vi "autoqueue.vi"(0 "cluster":T3, 1 "output cluster":T2, 3 "Cluster":cluster{"1":bool, "2":bool}, 4 "Report Data.Degree":dbl[][](array[numeric]), 5 "1to4":T1, 6 "milliseconds to wait":u32=100, 7 "path?":bool, 8 "milliseconds to wait 2":u32=100, 11 "error out":errorcluster, 12 "reference":refnum<vi>, 13 "Str Refnum":refnum<vi>, 14 "reference 2":refnum<vi>) -> (15 "error out 2":errorcluster)   [LabVIEW 2015]
uses:
  Typedef/Inst. Queue.ctl
  Typedef/State.ctl
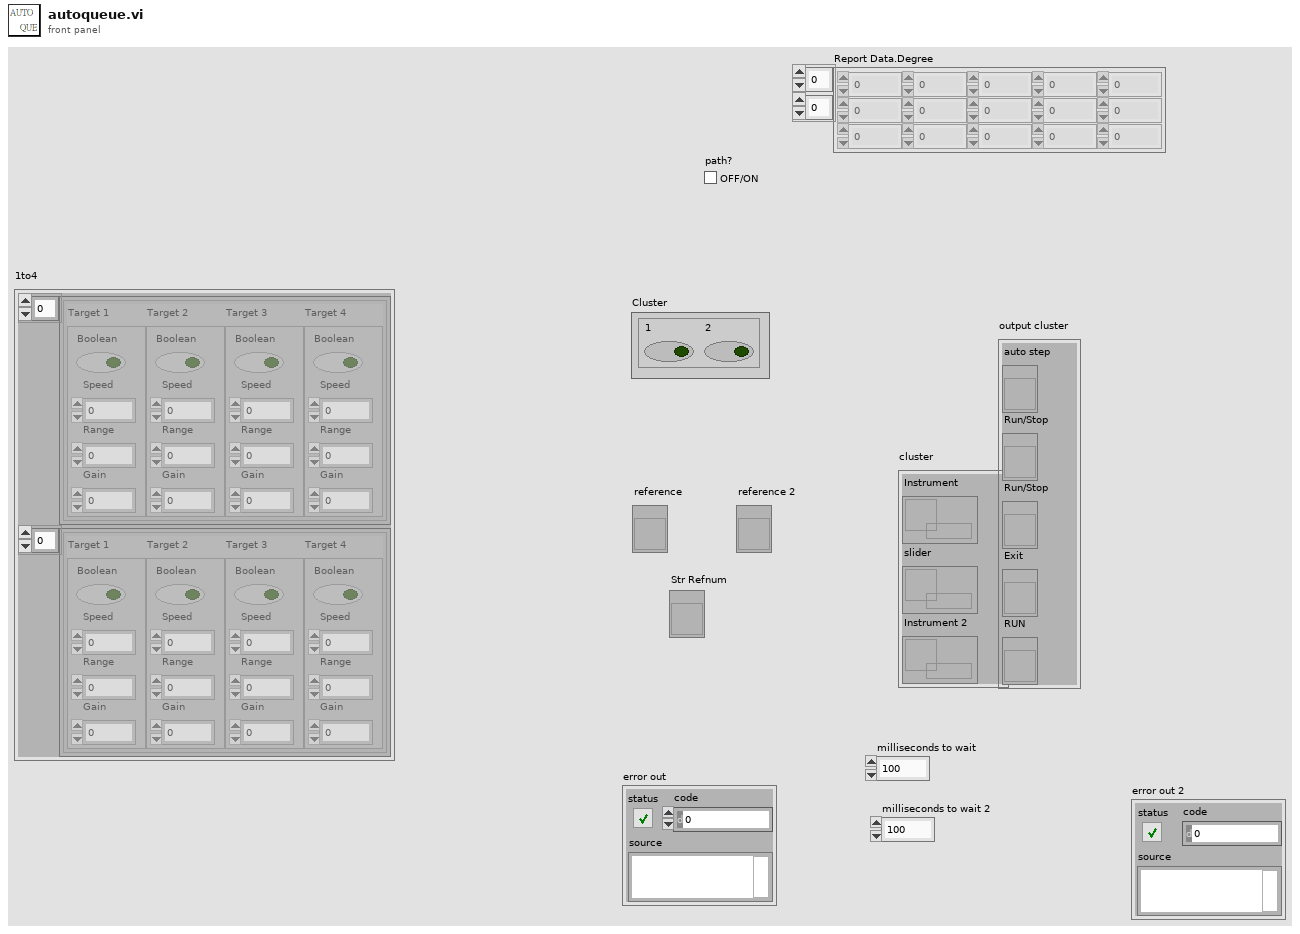
[diagram p1: front panel]
types:
  T1 = cluster{cluster{"Target 1":cluster{"Boolean":bool, "Speed":dbl, "Range":dbl, "Gain":dbl}, "Target 2":cluster{"Boolean":bool, "Speed":dbl, "Range":dbl, "Gain":dbl}, "Target 3":cluster{"Boolean":bool, "Speed":dbl, "Range":dbl, "Gain":dbl}, "Target 4":cluster{"Boolean":bool, "Speed":dbl, "Range":dbl, "Gain":dbl}}[], cluster{"Target 1":cluster{"Boolean":bool, "Speed":dbl, "Range":dbl, "Gain":dbl}, "Target 2":cluster{"Boolean":bool, "Speed":dbl, "Range":dbl, "Gain":dbl}, "Target 3":cluster{"Boolean":bool, "Speed":dbl, "Range":dbl, "Gain":dbl}, "Target 4":cluster{"Boolean":bool, "Speed":dbl, "Range":dbl, "Gain":dbl}}[]}
  T2 = cluster{"auto step":refnum<vi>, "Run/Stop":refnum<vi>, "Run/Stop":refnum<vi>, "Exit":refnum<vi>, "RUN":refnum<vi>}
  T3 = cluster{"Instrument":refnum<queue>, "slider":refnum<queue>, "Instrument 2":refnum<queue>}
  T4 = typedef "Inst. Queue.ctl" = cluster{enum16{"auto mode", "Idle", "Inst. Connect", "£m Data", "Inst. Update", "Freq. (GHz)", "rx att", "GTX (dB)", "GRX (dB)", "Range Trim(m)", "Gain Trim (dB)", "Distance to RUT", "Mapping", "Convert", "RF ON/OFF", "Run", "Direct Program", "Stop", "Dynamic", "dyset", "Exit"}, "variant":variant}
  T5 = cluster{"Target 1":cluster{"Boolean":bool, "Speed":dbl, "Range":dbl, "Gain":dbl}, "Target 2":cluster{"Boolean":bool, "Speed":dbl, "Range":dbl, "Gain":dbl}, "Target 3":cluster{"Boolean":bool, "Speed":dbl, "Range":dbl, "Gain":dbl}, "Target 4":cluster{"Boolean":bool, "Speed":dbl, "Range":dbl, "Gain":dbl}}[]
  T6 = typedef "State.ctl" = enum16{"Idle", "Initial", "Update", "get angle", "Axis", "Connect", "Creep", "Speed", "Distance", "Move Method", "Move Mode", "Direct of Movement", "Initail Speed", "Sramp", "Normal Open", "Acceleration", "Deceleration", "Angle", "Move&Rotate", "Rotate", "Rotate_2", "Return to Origin", "Move", "Inching", "Return to Zero", "Return to Middle", "Go to Step1", "Go to Step2", "Go to Step3", "Initial to Y Step", "Select Speed", "auto mode", "Stop", "reset xy", "reset ant", "set speed", "Exit"}
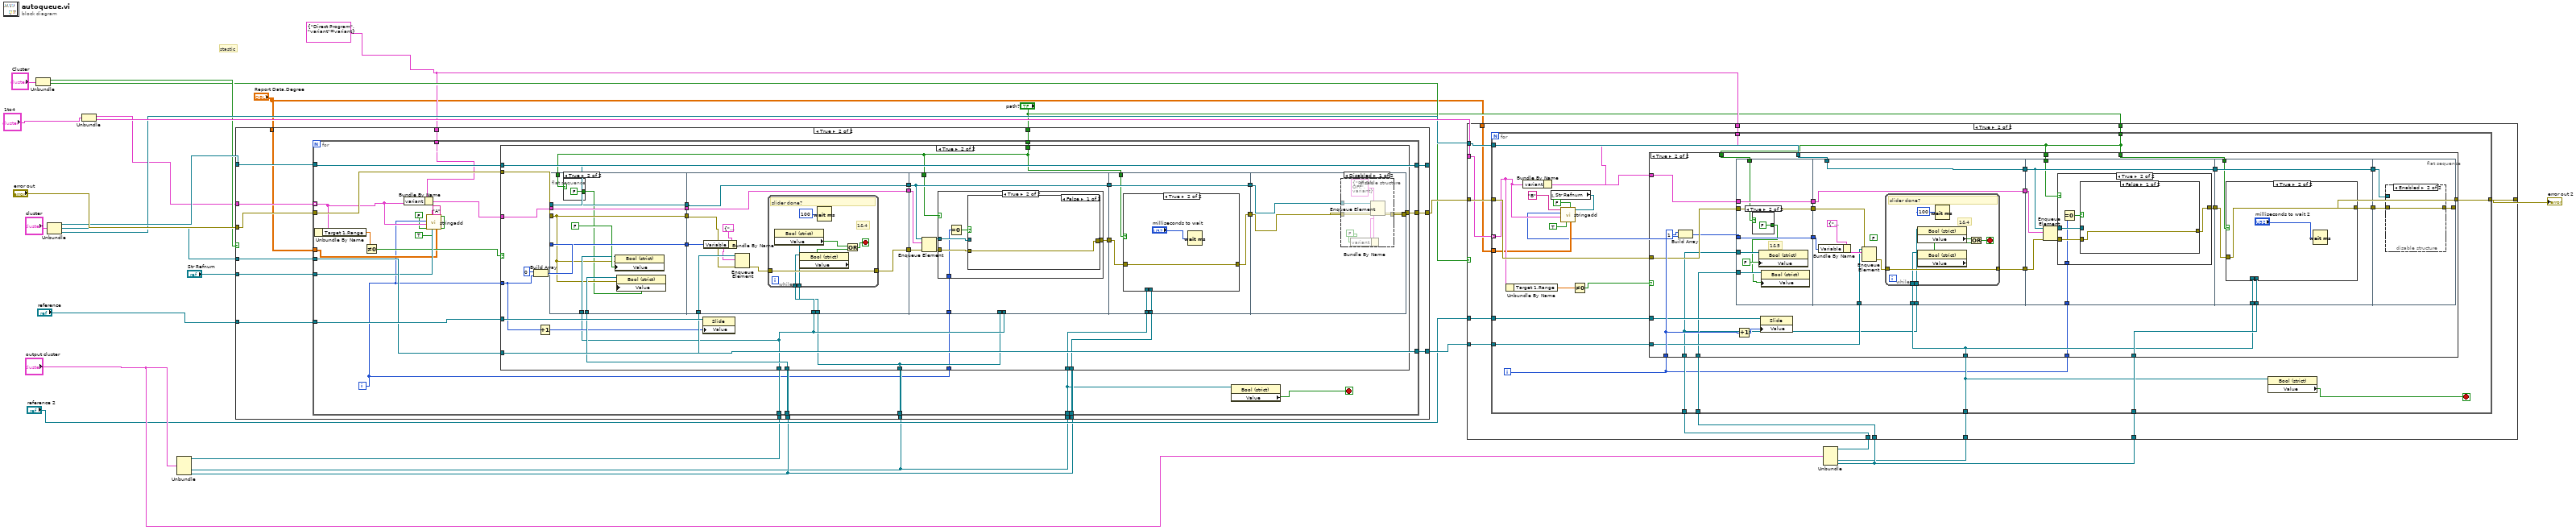
[diagram p0: block diagram]
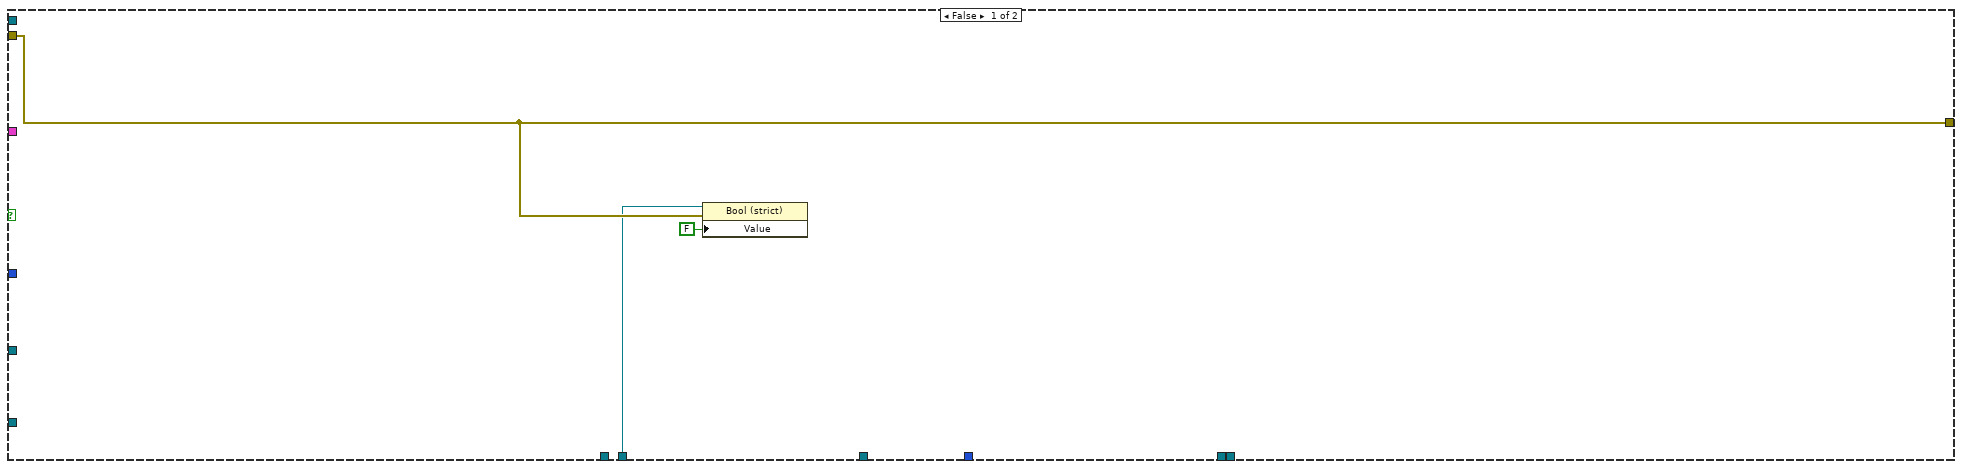
[diagram p3: hidden frame]
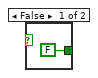
[diagram p4: hidden frame]
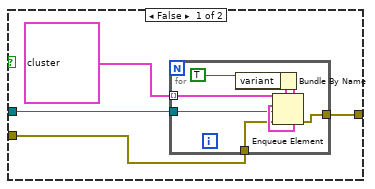
[diagram p5: hidden frame]
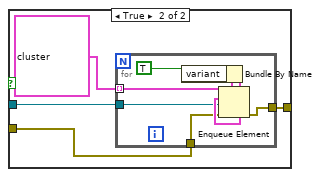
[diagram p6: hidden frame]
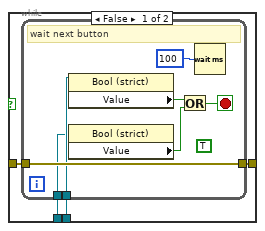
[diagram p7: hidden frame]
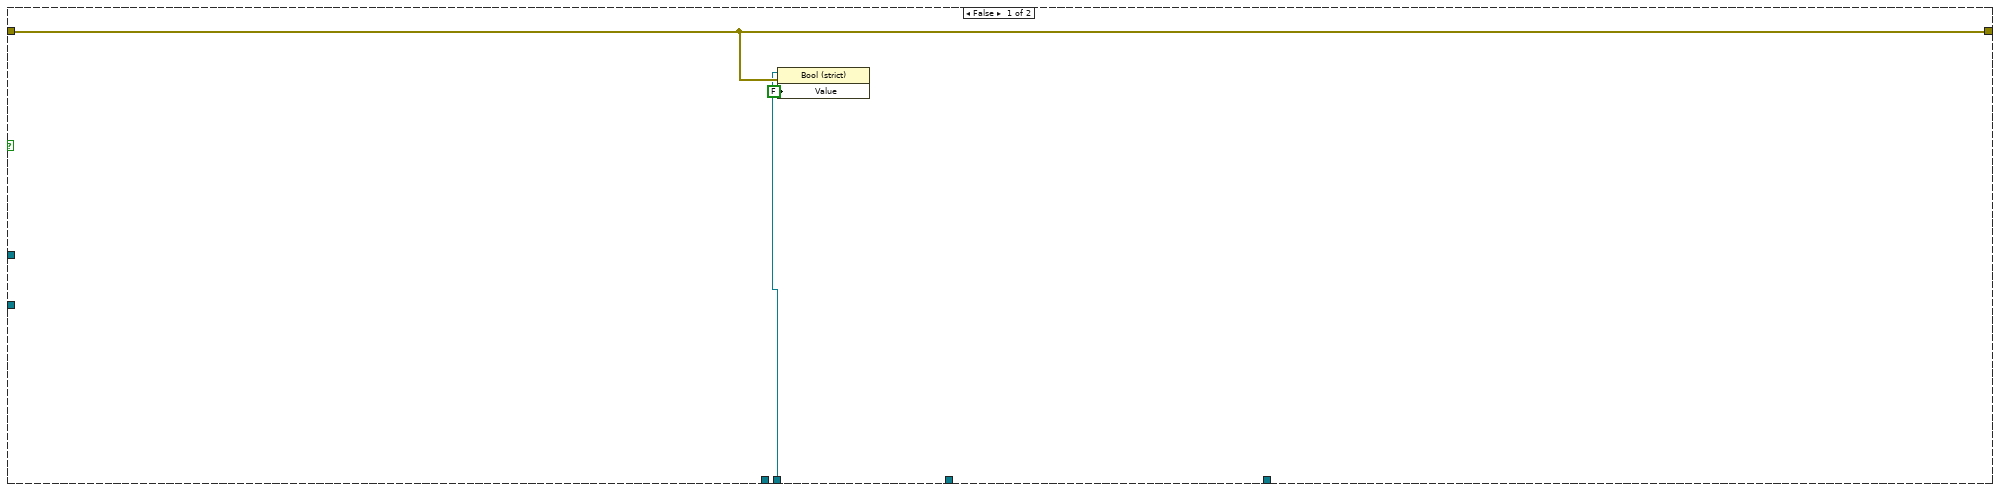
[diagram p9: hidden frame]
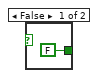
[diagram p11: hidden frame]
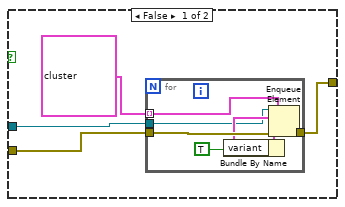
[diagram p12: hidden frame]
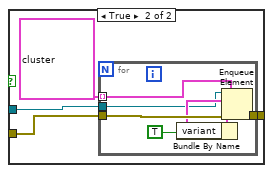
[diagram p13: hidden frame]
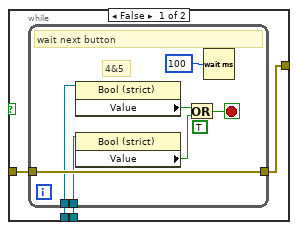
[diagram p14: hidden frame]
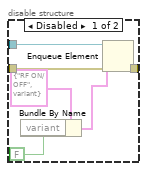
[diagram p15: hidden frame]
diagram:
  w5 = T4 {enum."Direct Program", "variant"=variant}
  # "stastic"
  n1 = Unbundle("Cluster") -> ("1"=w7:bool, "2"=w6:bool)
  n2 = Unbundle("cluster") -> ("Instrument"=w25:refnum<queue>, "slider"=w24:refnum<queue>, "Instrument 2"=w15:refnum<queue>)
  n3 = Unbundle("1to4") -> (w4:T5, w20:T5)
  n4 = Unbundle("output cluster") -> ("auto step"=w12:refnum<vi>, "Exit"=w11:refnum<vi>, "RUN"=w13:refnum<vi>)  [unwired: 2 out]
  n5 = case shown="True" w7 {
    tunnel: "error out" -> [w30 w47]
    tunnel: w25 -> [w29 w46]
    tunnel: w24 -> [w28 w45]
    tunnel: [w30 w44] -> w23
    tunnel: w4 -> [_ w43]
    tunnel: "reference" -> [_ w42]
    tunnel: [w29 w41] -> _
    tunnel: [w28 w40] -> w17
    tunnel: w13 -> [_ w39]
    tunnel: w13 -> [_ w38]
    tunnel: w12 -> [_ w37]
    tunnel: w11 -> [_ w36]
    tunnel: w11 -> [_ w35]
    tunnel: w5 -> [_ w34]
    tunnel: "Str Refnum" -> [_ w33]
    tunnel: "path?" -> [_ w32]
    tunnel: "Report Data.Degree" -> [_ w31]
    frame False {
    }
    frame True {
      n6 = for {
        tunnel: w46 -> [w67]
        tunnel: w43 -> [w56] mode=indexing
        tunnel: w45 -> [w66]
        tunnel: w42 -> [w68]
        tunnel: [w67] -> w41
        tunnel: [w66] -> w40
        tunnel: w39 -> [w58]
        tunnel: w38 -> [w65]
        tunnel: w37 -> [w59]
        tunnel: w36 -> [w64]
        tunnel: w35 -> [w61]
        tunnel: w34 -> [w63]
        tunnel: w33 -> [w62]
        tunnel: w47 -> [w69]
        tunnel: [w70] -> w44
        tunnel: w32 -> [w57]
        tunnel: w31 -> [w52]
        i -> [w51]
        stop <- w60 stop-if-true
        n7 = Unbundle By Name(w56) -> ("Target 1.Range"=w55:dbl)
        n8 = Not Equal To 0?(x=w55) -> (x != 0?=w53:bool)
        n9 = Bundle By Name(cluster=w63, "variant"=w56) -> (w54:T4)
        n10 = call "stringadd.vi"("Report Data.Degree"=w52, "Mode"=FALSE, "s/d setting"=TRUE, "Str Refnum"=w62, "variant"=w56, "Numeric"=w51, "String"="A") -> ()  [unwired: 5 in]
        n11 = case shown="True" w53 {
          tunnel: [w73 w92] -> w70
          tunnel: w69 -> [w73 w91]
          tunnel: w68 -> [_ w90]
          tunnel: w67 -> [_ w89]
          tunnel: w66 -> [_ w88]
          tunnel: w65 -> [_ w87]
          tunnel: w64 -> [_ w78]
          tunnel: w51 -> [_ w86]
          tunnel: w61 -> [_ w85]
          tunnel: w59 -> [_ w79]
          tunnel: w58 -> [w72 w84]
          tunnel: w57 -> [_ w75]
          tunnel: w54 -> [_ w83]
          tunnel: w51 -> [_ w74]
          frame False {
            n12 = property on="Property Node" class="Bool (strict)"(reference=w72, error in=w73, "Value"=FALSE) -> ()  [unwired: 2 out]
          }
          frame True {
            n13 = Build Array(0 ("element"), w86) -> (w80:i32[])
            n14 = Increment(x=w86) -> (x+1=w82:i32)
            n15 = flat-sequence {
              tunnel: w80 -> [w108]
              tunnel: w91 -> [w104]
              tunnel: w89 -> [w109]
              tunnel: w83 -> [w110]
              tunnel: [w110] -> w101
              tunnel: [w109] -> w100
              tunnel: [w108] -> w99
              tunnel: w79 -> [w106]
              tunnel: w84 -> [w105]
              tunnel: [w104] -> w98
              tunnel: w75 -> [w103]
              tunnel: w88 -> [w123]
              tunnel: [w114] -> w97
              tunnel: w101 -> [w115]
              tunnel: w100 -> [w114]
              tunnel: w99 -> [w121]
              tunnel: w98 -> [w113]
              tunnel: w79 -> [w118]
              tunnel: w78 -> [w117]
              tunnel: [w116] -> w77
              tunnel: [w115] -> w76
              tunnel: [w138] -> w96
              tunnel: [w134] -> w95
              tunnel: w97 -> [w134]
              tunnel: w79 -> [_]
              tunnel: w78 -> [_]
              tunnel: w77 -> [w137]
              tunnel: w76 -> [w135]
              tunnel: w75 -> [w132]
              tunnel: w74 -> [w131]
              tunnel: w96 -> [w170]
              tunnel: [w169] -> w94
              tunnel: [w168] -> w93
              tunnel: w95 -> [w168]
              tunnel: w87 -> [w167]
              tunnel: w85 -> [w166]
              tunnel: w75 -> [w165]
              tunnel: [w186] -> w92
              tunnel: w94 -> [w184]
              tunnel: w93 -> [w185]
              frame #0 {
                n16 = case shown="True" w103 {
                  tunnel: [FALSE FALSE] -> w102
                  frame False {
                  }
                  frame True {
                  }
                }
                n17 = property on="Property Node" class="Bool (strict)"(reference=w106, error in=w104, "Value"=FALSE) -> ()  [unwired: 2 out]
                n18 = property on="Property Node" class="Bool (strict)"(reference=w105, error in=w104, "Value"=w102) -> ()  [unwired: 2 out]
              }
              frame #1 {
                n19 = Bundle By Name(cluster=cluster{"State":T6, "Variable":variant} {"State"=enum."auto mode", "Variable"=variant}, "Variable"=w121) -> (w120:cluster{"State":T6, "Variable":variant})
                n20 = Enqueue Element(queue=w123, element=w120, error in (no error)=w113) -> (error out=w119:errorcluster)  [unwired: 1 in, 2 out]
                n21 = while {
                  tunnel: w119 -> [w130]
                  tunnel: [w130] -> w116
                  tunnel: w117 -> [w125]
                  tunnel: w118 -> [w124]
                  stop <- w126 stop-if-true
                  # "1&4"
                  # "slider done?"
                  n22 = property on="Property Node" class="Bool (strict)"(reference=w125) -> ("Value"=w128:bool)  [unwired: 1 in, 2 out]
                  n23 = property on="Property Node" class="Bool (strict)"(reference=w124) -> ("Value"=w127:bool)  [unwired: 1 in, 2 out]
                  n24 = Wait (ms)(milliseconds to wait=u32 100) -> ()  [unwired: 1 out]
                  n25 = Or(x=w128, y=w127) -> (x .or. y?=w126:bool)
                }
              }
              frame #2 {
                n26 = Enqueue Element(queue=w134, element=w135, error in (no error)=w137) -> (queue out=w133:refnum<queue>, error out=w136:errorcluster)  [unwired: 1 in, 1 out]
                n27 = case shown="True" w132 {
                  tunnel: [w142 w153] -> w138
                  tunnel: w136 -> [w141 w152]
                  tunnel: w133 -> [w140 w151]
                  tunnel: w131 -> [_ w150]
                  frame False {
                    n28 = for {
                      tunnel: T4[] [{enum."Convert", "variant"=variant}, {enum."RF ON/OFF", "variant"=variant}] -> [w147] mode=indexing
                      tunnel: [w148] -> w142
                      tunnel: w141 -> [w144]
                      tunnel: w140 -> [w143]
                      n29 = Bundle By Name(cluster=w147, "variant"=TRUE) -> (w146:T4)
                      n30 = Enqueue Element(queue=w143, element=w146, error in (no error)=w144) -> (error out=w148:errorcluster)  [unwired: 1 in, 2 out]
                    }
                  }
                  frame True {
                    n31 = Equal To 0?(x=w150) -> (x = 0?=w149:bool)
                    n32 = case shown="False" w149 {
                      tunnel: [w154 w158] -> w153
                      tunnel: w152 -> [w154 w157]
                      tunnel: w151 -> [_ w156]
                      frame False {
                      }
                      frame True {
                        n33 = for {
                          tunnel: T4[] [{enum."Convert", "variant"=variant}, {enum."RF ON/OFF", "variant"=variant}] -> [w163] mode=indexing
                          tunnel: [w164] -> w158
                          tunnel: w157 -> [w160]
                          tunnel: w156 -> [w159]
                          n34 = Bundle By Name(cluster=w163, "variant"=TRUE) -> (w162:T4)
                          n35 = Enqueue Element(queue=w159, element=w162, error in (no error)=w160) -> (error out=w164:errorcluster)  [unwired: 1 in, 2 out]
                        }
                      }
                    }
                  }
                }
              }
              frame #3 {
                n36 = case shown="True" w165 {
                  tunnel: w170 -> [w174 w183]
                  tunnel: [w173 w183] -> w169
                  tunnel: w167 -> [w172 _]
                  tunnel: w166 -> [w171 _]
                  frame False {
                    n37 = while {
                      tunnel: w174 -> [w180]
                      tunnel: [w180] -> w173
                      tunnel: w172 -> [w177]
                      tunnel: w171 -> [w176]
                      stop <- w175 stop-if-true
                      (unwired) TRUE
                      # "wait next button"
                      n38 = property on="Property Node" class="Bool (strict)"(reference=w177) -> ("Value"=w179:bool)  [unwired: 1 in, 2 out]
                      n39 = property on="Property Node" class="Bool (strict)"(reference=w176) -> ("Value"=w178:bool)  [unwired: 1 in, 2 out]
                      n40 = Or(x=w179, y=w178) -> (x .or. y?=w175:bool)
                      n41 = Wait (ms)(milliseconds to wait=u32 100) -> ()  [unwired: 1 out]
                    }
                  }
                  frame True {
                    n42 = Wait (ms)(milliseconds to wait="milliseconds to wait") -> ()  [unwired: 1 out]
                  }
                }
              }
              frame #4 {
                n43 = disable-structure shown="Disabled" {
                  disable-tunnel: [w192 w193] -> w186
                  disable-tunnel: w184 -> [w188 w193]
                  disable-tunnel: w185 -> [w187 _]
                  frame Disabled {
                    n44 = Bundle By Name(cluster=T4 {enum."RF ON/OFF", "variant"=variant}, "variant"=FALSE) -> (w190:T4)
                    n45 = Enqueue Element(queue=w187, element=w190, error in (no error)=w188) -> (error out=w192:errorcluster)  [unwired: 1 in, 2 out]
                  }
                  frame Enabled {
                  }
                }
              }
            }
            n46 = property class="Slide"(reference=w90, "Value"=w82) -> ()  [unwired: 1 in, 2 out]
          }
        }
        n47 = property on="Property Node" class="Bool (strict)"(reference=w61) -> ("Value"=w60:bool)  [unwired: 1 in, 2 out]
      }
    }
  }
  n48 = Unbundle("output cluster") -> ("auto step"=w10:refnum<vi>, "Exit"=w8:refnum<vi>, "RUN"=w9:refnum<vi>)  [unwired: 2 out]
  n49 = case shown="True" w6 {
    tunnel: w23 -> [w196 w209]
    tunnel: [w196 w208] -> w22
    tunnel: w20 -> [_ w198]
    tunnel: "reference 2" -> [_ w207]
    tunnel: w15 -> [_ w206]
    tunnel: w17 -> [_ w205]
    tunnel: w10 -> [_ w204]
    tunnel: w9 -> [w195 w203]
    tunnel: w9 -> [_ w202]
    tunnel: w8 -> [_ w201]
    tunnel: w5 -> [_ w200]
    tunnel: "path?" -> [_ w199]
    tunnel: "Report Data.Degree" -> [_ w197]
    frame False {
      n50 = property on="Property Node" class="Bool (strict)"(reference=w195, error in=w196, "Value"=FALSE) -> ()  [unwired: 2 out]
    }
    frame True {
      n51 = for {
        tunnel: w198 -> [w219] mode=indexing
        tunnel: w207 -> [w228]
        tunnel: w206 -> [w226]
        tunnel: w205 -> [w227]
        tunnel: w204 -> [w221]
        tunnel: w203 -> [w222]
        tunnel: w202 -> [w224]
        tunnel: w201 -> [w220]
        tunnel: w200 -> [w225]
        tunnel: w209 -> [w229]
        tunnel: [w230] -> w208
        tunnel: w199 -> [w215]
        tunnel: w197 -> [w216]
        i -> [w214]
        stop <- w223 stop-if-true
        n52 = Unbundle By Name(w219) -> ("Target 1.Range"=w218:dbl)
        n53 = Bundle By Name(cluster=w225, "variant"=w219) -> (w231:T4)
        n54 = local read "Str Refnum"() -> (w212:refnum<vi>)
        n55 = call "stringadd.vi"("Report Data.Degree"=w216, "Mode"=FALSE, "s/d setting"=TRUE, "Str Refnum"=w212, "variant"=w219, "Numeric"=w214, "String"="B") -> ()  [unwired: 5 in]
        n56 = Not Equal To 0?(x=w218) -> (x != 0?=w217:bool)
        n57 = case shown="True" w217 {
          tunnel: w231 -> [_ w252]
          tunnel: [w232 w251] -> w230
          tunnel: w229 -> [w232 w250]
          tunnel: w228 -> [_ w249]
          tunnel: w227 -> [_ w248]
          tunnel: w226 -> [_ w247]
          tunnel: w214 -> [_ w243]
          tunnel: w224 -> [_ w242]
          tunnel: w222 -> [_ w241]
          tunnel: w221 -> [_ w237]
          tunnel: w215 -> [_ w240]
          tunnel: w220 -> [_ w238]
          tunnel: w215 -> [_ w239]
          tunnel: w215 -> [_ w234]
          tunnel: w214 -> [_ w233]
          frame False {
          }
          frame True {
            n58 = Build Array(1 ("element"), w243) -> (w245:i32[])
            n59 = flat-sequence {
              tunnel: w245 -> [w266]
              tunnel: w250 -> [w267]
              tunnel: w252 -> [w268]
              tunnel: [w268] -> w260
              tunnel: [w267] -> w259
              tunnel: [w266] -> w258
              tunnel: w241 -> [w265]
              tunnel: w237 -> [w264]
              tunnel: w239 -> [w261]
              tunnel: [w276] -> w257
              tunnel: w248 -> [w277]
              tunnel: w247 -> [w276]
              tunnel: w260 -> [w271]
              tunnel: w259 -> [w278]
              tunnel: w258 -> [w280]
              tunnel: w238 -> [w274]
              tunnel: w237 -> [w273]
              tunnel: [w272] -> w236
              tunnel: [w271] -> w235
              tunnel: [w296] -> w256
              tunnel: [w295] -> w255
              tunnel: w257 -> [w295]
              tunnel: w236 -> [w293]
              tunnel: w235 -> [w291]
              tunnel: w234 -> [w290]
              tunnel: w233 -> [w289]
              tunnel: w256 -> [w328]
              tunnel: [w327] -> w254
              tunnel: [w326] -> w253
              tunnel: w255 -> [w326]
              tunnel: w242 -> [w325]
              tunnel: w238 -> [w324]
              tunnel: w240 -> [w323]
              tunnel: [w344] -> w251
              tunnel: w254 -> [w343]
              tunnel: w253 -> [w342]
              frame #0 {
                # "1&5"
                n60 = case shown="True" w261 {
                  tunnel: [FALSE FALSE] -> w262
                  frame False {
                  }
                  frame True {
                  }
                }
                n61 = property on="Property Node" class="Bool (strict)"(reference=w264, "Value"=FALSE) -> ()  [unwired: 1 in, 2 out]
                n62 = property on="Property Node" class="Bool (strict)"(reference=w265, "Value"=w262) -> ()  [unwired: 1 in, 2 out]
              }
              frame #1 {
                (unwired) FALSE ("Value")
                n63 = Bundle By Name(cluster=cluster{"State":T6, "Variable":variant} {"State"=enum."auto mode", "Variable"=variant}, "Variable"=w280) -> (w279:cluster{"State":T6, "Variable":variant})
                n64 = Enqueue Element(queue=w277, element=w279, error in (no error)=w278) -> (error out=w275:errorcluster)  [unwired: 1 in, 2 out]
                n65 = while {
                  tunnel: w275 -> [w288]
                  tunnel: [w288] -> w272
                  tunnel: w273 -> [w283]
                  tunnel: w274 -> [w282]
                  stop <- w284 stop-if-true
                  # "1&4"
                  # "slider done?"
                  n66 = property on="Property Node" class="Bool (strict)"(reference=w283) -> ("Value"=w286:bool)  [unwired: 1 in, 2 out]
                  n67 = property on="Property Node" class="Bool (strict)"(reference=w282) -> ("Value"=w285:bool)  [unwired: 1 in, 2 out]
                  n68 = Wait (ms)(milliseconds to wait=u32 100) -> ()  [unwired: 1 out]
                  n69 = Or(x=w286, y=w285) -> (x .or. y?=w284:bool)
                }
              }
              frame #2 {
                n70 = Enqueue Element(queue=w295, element=w291, error in (no error)=w293) -> (queue out=w294:refnum<queue>, error out=w292:errorcluster)  [unwired: 1 in, 1 out]
                n71 = case shown="True" w290 {
                  tunnel: [w300 w311] -> w296
                  tunnel: w294 -> [w299 w310]
                  tunnel: w292 -> [w298 w309]
                  tunnel: w289 -> [_ w308]
                  frame False {
                    n72 = for {
                      tunnel: T4[] [{enum."Convert", "variant"=variant}, {enum."RF ON/OFF", "variant"=variant}] -> [w304] mode=indexing
                      tunnel: w298 -> [w306]
                      tunnel: [w305] -> w300
                      tunnel: w299 -> [w301]
                      n73 = Bundle By Name(cluster=w304, "variant"=TRUE) -> (w303:T4)
                      n74 = Enqueue Element(queue=w301, element=w303, error in (no error)=w306) -> (error out=w305:errorcluster)  [unwired: 1 in, 2 out]
                    }
                  }
                  frame True {
                    n75 = Equal To 0?(x=w308) -> (x = 0?=w307:bool)
                    n76 = case shown="False" w307 {
                      tunnel: [w312 w316] -> w311
                      tunnel: w310 -> [_ w315]
                      tunnel: w309 -> [w312 w314]
                      frame False {
                      }
                      frame True {
                        n77 = for {
                          tunnel: T4[] [{enum."Convert", "variant"=variant}, {enum."RF ON/OFF", "variant"=variant}] -> [w320] mode=indexing
                          tunnel: w314 -> [w322]
                          tunnel: [w321] -> w316
                          tunnel: w315 -> [w317]
                          n78 = Bundle By Name(cluster=w320, "variant"=TRUE) -> (w319:T4)
                          n79 = Enqueue Element(queue=w317, element=w319, error in (no error)=w322) -> (error out=w321:errorcluster)  [unwired: 1 in, 2 out]
                        }
                      }
                    }
                  }
                }
              }
              frame #3 {
                n80 = case shown="True" w323 {
                  tunnel: w328 -> [w332 w341]
                  tunnel: [w331 w341] -> w327
                  tunnel: w325 -> [w330 _]
                  tunnel: w324 -> [w329 _]
                  frame False {
                    n81 = while {
                      tunnel: w332 -> [w338]
                      tunnel: [w338] -> w331
                      tunnel: w330 -> [w335]
                      tunnel: w329 -> [w334]
                      stop <- w333 stop-if-true
                      (unwired) TRUE
                      # "4&5"
                      # "wait next button"
                      n82 = property on="Property Node" class="Bool (strict)"(reference=w334) -> ("Value"=w337:bool)  [unwired: 1 in, 2 out]
                      n83 = property on="Property Node" class="Bool (strict)"(reference=w335) -> ("Value"=w336:bool)  [unwired: 1 in, 2 out]
                      n84 = Or(x=w337, y=w336) -> (x .or. y?=w333:bool)
                      n85 = Wait (ms)(milliseconds to wait=u32 100) -> ()  [unwired: 1 out]
                    }
                  }
                  frame True {
                    n86 = Wait (ms)(milliseconds to wait="milliseconds to wait 2") -> ()  [unwired: 1 out]
                  }
                }
              }
              frame #4 {
                n87 = disable-structure shown="Enabled" {
                  disable-tunnel: [w350 w351] -> w344
                  disable-tunnel: w343 -> [w349 w351]
                  disable-tunnel: w342 -> [w345 _]
                  frame Disabled {
                    n88 = Bundle By Name(cluster=T4 {enum."RF ON/OFF", "variant"=variant}, "variant"=FALSE) -> (w347:T4)
                    n89 = Enqueue Element(queue=w345, element=w347, error in (no error)=w349) -> (error out=w350:errorcluster)  [unwired: 1 in, 2 out]
                  }
                  frame Enabled {
                  }
                }
              }
            }
            n90 = Increment(x=w243) -> (x+1=w246:i32)
            n91 = property class="Slide"(reference=w249, "Value"=w246) -> ()  [unwired: 1 in, 2 out]
          }
        }
        n92 = property on="Property Node" class="Bool (strict)"(reference=w220) -> ("Value"=w223:bool)  [unwired: 1 in, 2 out]
      }
    }
  }
  "error out 2" <- w22
